vi "Get Chan Data for typedefs.vi"(7 "Custom Device Ref":T1=18446744073709551615 format="%.0x", 8 "error in":errorcluster, 10 "Ctl Ref":refnum<vi>, 11 "Section Ref in":T1 format="%.0x") -> (0 "error out":errorcluster, 2 "Indexes":i32[](array[numeric]), 3 "Section Ref out":T1 format="%.0x")   [LabVIEW 2016, in "DCM System Explorer.lvlib"]
uses:
  DCM System Explorer.lvlib
  <vilib>/NI Veristand/Custom Device API/Custom Device Item Ref.ctl
  <vilib>/NI VeriStand/Custom Device API/Custom Device API.lvlib
  <vilib>/NI Veristand/Custom Device Tools/Custom Device Utility Library/Custom Device Utility Library.lvlib
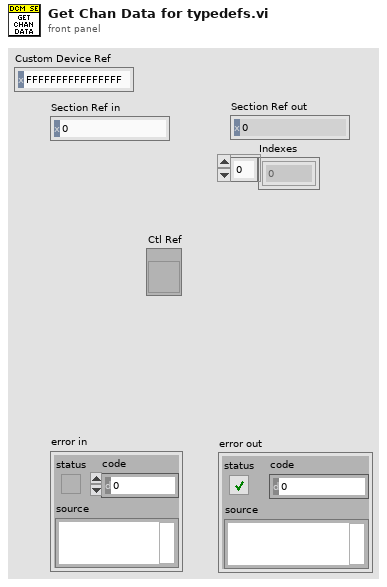
[diagram p1: front panel]
types:
  T1 = typedef "Custom Device API.lvlib/Custom Device Item Ref.ctl" = u64
  T2 = cluster{"Index Ref":refnum<vi>, "Array Refs":refnum<vi>[], "Array Positions":i32[][], "Device Ref":T1, "Section Ref":T1, "GUIDChDelProt":string, "GUIDSectDelProt":string}
  T3 = cluster{"Index Ref":refnum<vi>, "Array Refs":refnum<vi>[], "Array Positions":i32[][], "Device Ref":T1, "Section Ref":T1, "GUIDChDelProt":string, "GUIDSectDelProt":string}[]
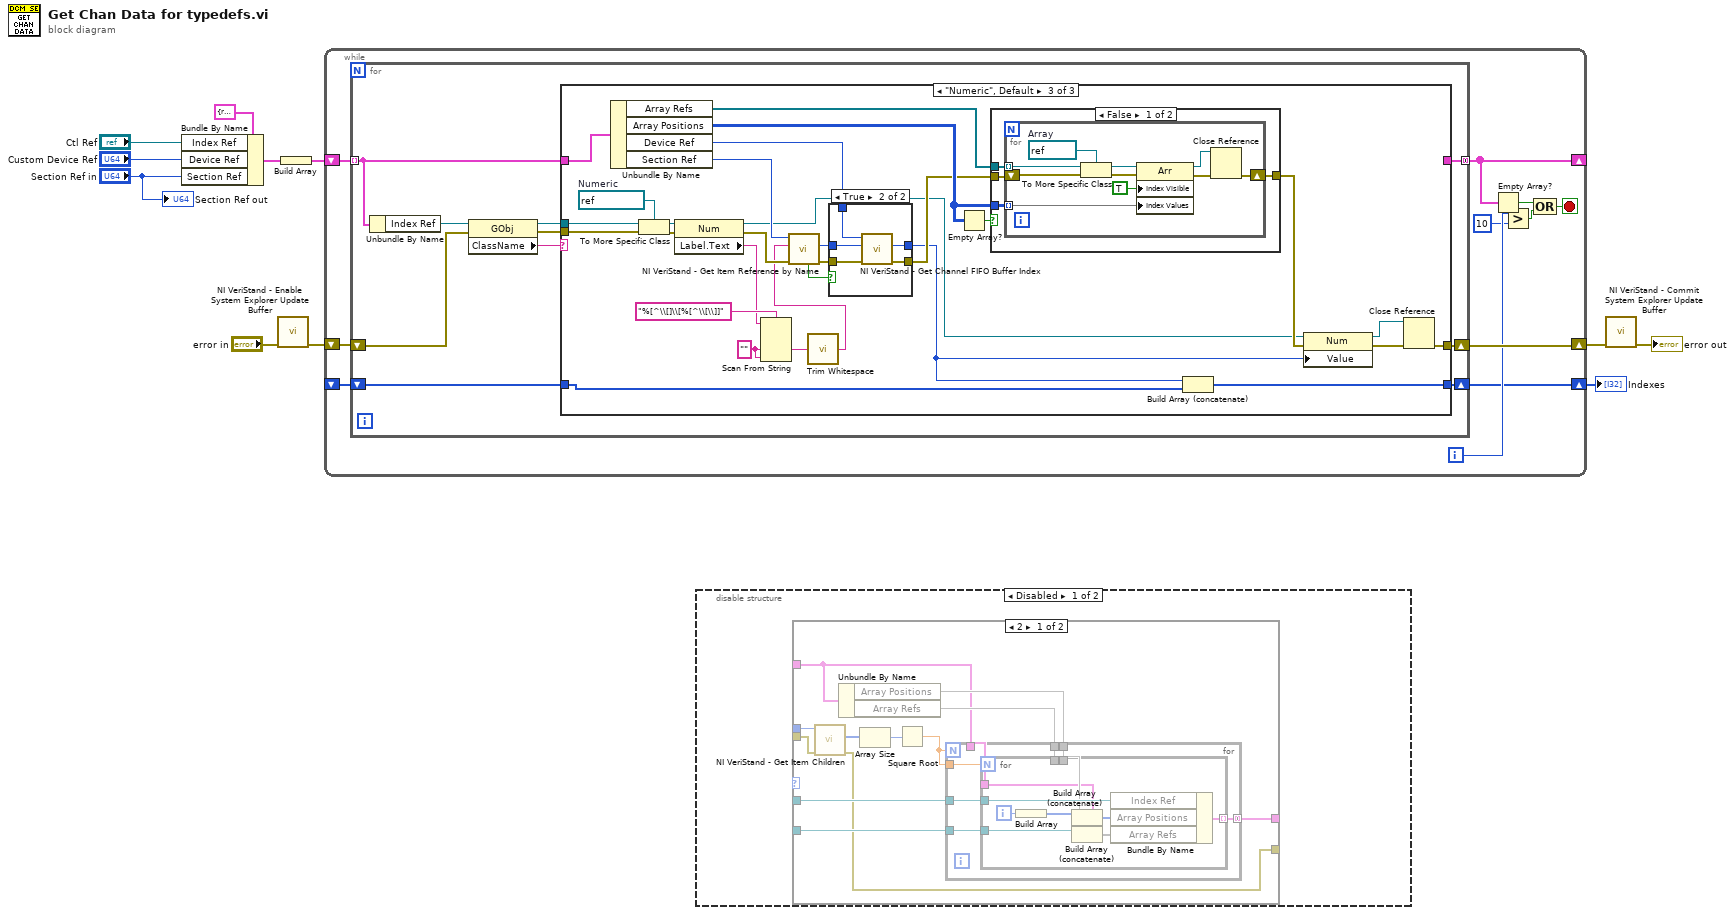
[diagram p0: block diagram]
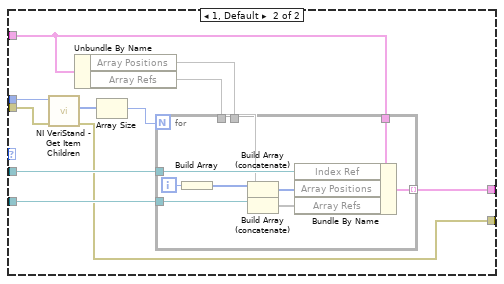
[diagram p2: hidden frame]
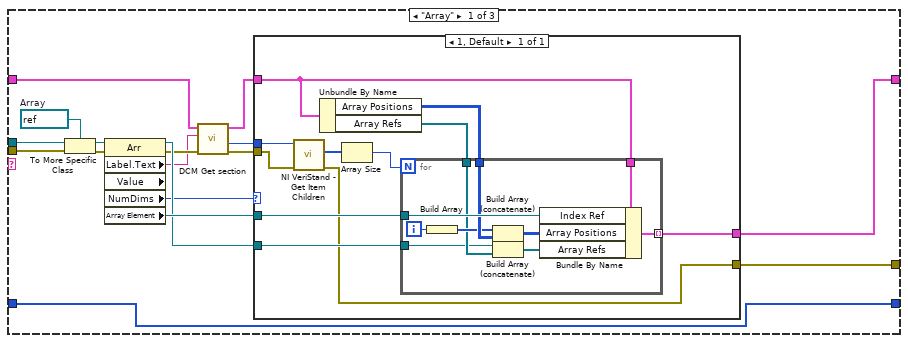
[diagram p4: hidden frame]
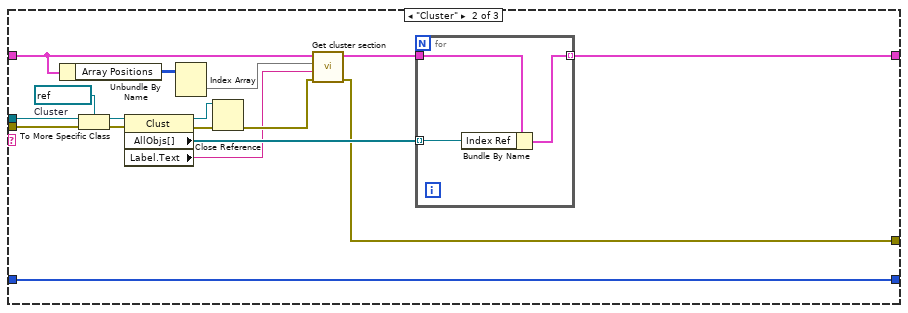
[diagram p5: hidden frame]
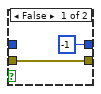
[diagram p6: hidden frame]
diagram:
  n1 = Bundle By Name(cluster=T2 {"Index Ref"=refnum, "Array Refs"=[], "Array Positions"=[], "Device Ref"=0, "Section Ref"=0, "GUIDChDelProt"="", "GUIDSectDelProt"=""} ("Data"), "Index Ref"="Ctl Ref", "Device Ref"="Custom Device Ref", "Section Ref"="Section Ref in") -> (w10:T2)
  n2 = call <vilib>:"NI VeriStand - Enable System Explorer Update Buffer.vi"("error in (no error)"="error in") -> ("error out"=w2:errorcluster)  [unwired: 10 in]
  n3 = Build Array(w10) -> (w11:T3)
  n4 = while {
    shift-right: [w21] -> _
    shift-left: w11 -> [w22]
    shift-right: [w20] -> w5
    shift-left: w2 -> [w19]
    shift-right: [w13] -> w1
    shift-left: _ -> [w12]
    i -> [w16]
    stop <- w17 stop-if-true
    n5 = for {
      tunnel: w22 -> [w29] mode=indexing
      tunnel: [w25] -> w21 mode=concatenating
      shift-right: [w30] -> w20
      shift-left: w19 -> [w26]
      shift-right: [w24] -> w13
      shift-left: w12 -> [w23]
      n6 = Unbundle By Name(w29) -> ("Index Ref"=w31:refnum<vi>)
      n7 = property class="GObj"(reference=w31, error in=w26) -> (reference out=w32:refnum<vi>, error out=w27:errorcluster, "ClassName"=w28:string)
      n8 = case shown="\"Numeric\", Default" w28 {
        tunnel: w32 -> [w49 w85 w119]
        tunnel: w27 -> [w46 w84 w117]
        tunnel: [w43 w73 w105] -> w30
        tunnel: w29 -> [w41 w77 w116]
        tunnel: [w44 w78 _] -> w25
        tunnel: [w33 w71 w91] -> w24
        tunnel: w23 -> [w33 w71 w92]
        frame "Array" {
          w45 = refnum<vi> refnum  # Array
          n9 = To More Specific Class(target class=w45, reference=w49, error in=w46) -> (specific class reference=w48:refnum<vi>, error out=w47:errorcluster)
          n10 = property class="Arr" props=["Label", "Text", "Value", "NumDims", "Array Element"](reference=w48, error in=w47) -> (reference out=w38:refnum<vi>, error out=w37:errorcluster, "Label.Text"=w36:string, "NumDims"=w34:u32, "Array Element"=w42:refnum<vi>)  [unwired: 1 out]
          n11 = call "DCM Get section.vi"("error in"=w37, "Label.Text in"=w36, "Data in"=w41) -> ("error out"=w39:errorcluster, "Section Ptr"=w35:T1, "Data out"=w40:T2)  [unwired: 6 in]
          n12 = case shown="1, Default" w34 {
            tunnel: w39 -> [w50]
            tunnel: w40 -> [w56]
            tunnel: [w60] -> w44
            tunnel: [w53] -> w43
            tunnel: w42 -> [w59]
            tunnel: w38 -> [w55]
            tunnel: w35 -> [w51]
            frame 1, Default {
              n13 = call <vilib>:"NI VeriStand - Get Item Children.vi"("error in (no error)"=w50, "Item Ref in"=w51) -> ("error out"=w53:errorcluster, "Child Refs"=w54:T1[])  [unwired: 6 in, 2 out]
              n14 = Unbundle By Name(w56) -> ("Array Positions"=w58:i32[][], "Array Refs"=w57:refnum<vi>[])
              n15 = Array Size(array=w54) -> (size(s)=w52:i32)
              n16 = for {
                N: w52 -> [_]
                tunnel: w56 -> [w70]
                tunnel: [w69] -> w60 mode=indexing
                tunnel: w59 -> [w67]
                tunnel: w55 -> [w61]
                tunnel: w58 -> [w64]
                tunnel: w57 -> [w62]
                i -> [w68]
                n17 = Build Array(w68) -> (w63:i32[])
                n18 = Build Array (concatenate)(w63, w64) -> (w66:i32[][])
                n19 = Build Array (concatenate)(w61, w62) -> (w65:refnum<vi>[])
                n20 = Bundle By Name(cluster=w70, "Index Ref"=w67, "Array Positions"=w66, "Array Refs"=w65) -> (w69:T2)
              }
            }
          }
        }
        frame "Cluster" {
          w83 = refnum<vi> refnum  # Cluster
          n21 = Unbundle By Name(w77) -> ("Array Positions"=w81:i32[][])
          n22 = To More Specific Class(target class=w83, reference=w85, error in=w84) -> (specific class reference=w87:refnum<vi>, error out=w86:errorcluster)
          n23 = property class="Clust"(reference=w87, error in=w86) -> (reference out=w80:refnum<vi>, error out=w79:errorcluster, "AllObjs[]"=w82:refnum<vi>[], "Label.Text"=w72:string)
          n24 = Index Array(array=w81) -> (element=w76:i32[])  [unwired: 2 in]
          n25 = Close Reference(reference=w80, error in (no error)=w79) -> (error out=w74:errorcluster)
          n26 = call "Get cluster section.vi"("error in (no error)"=w74, "Name (none)"=w72, "Array Positions (none)"=w76, "Data in"=w77) -> ("error out"=w73:errorcluster, "Data out"=w75:T2)  [unwired: 4 in, 2 out]
          n27 = for {
            tunnel: w75 -> [w89]
            tunnel: w82 -> [w88] mode=indexing
            tunnel: [w90] -> w78 mode=indexing
            n28 = Bundle By Name(cluster=w89, "Index Ref"=w88) -> (w90:T2)
          }
        }
        frame "Numeric", Default {
          w104 = "" ("default value 2")
          w114 = refnum<vi> refnum  # Numeric
          n29 = Unbundle By Name(w116) -> ("Array Refs"=w112:refnum<vi>[], "Array Positions"=w110:i32[][], "Device Ref"=w115:T1, "Section Ref"=w101:T1)
          n30 = To More Specific Class(target class=w114, reference=w119, error in=w117) -> (specific class reference=w118:refnum<vi>, error out=w113:errorcluster)
          n31 = property class="Num"(reference=w118, error in=w113) -> (reference out=w95:refnum<vi>, error out=w100:errorcluster, "Label.Text"=w94:string)
          n32 = Scan From String(format string="%[^\\[]\\[%[^\\[\\]]" ("regular expression"), input string=w94, default 1=w104, default 2=w104) -> (output 1=w103:string)  [unwired: 3 in, 3 out]
          n33 = call <vilib>:"Trim Whitespace.vi"("string"=w103) -> ("trimmed string"=w97:string)  [unwired: 1 in]
          n34 = call <vilib>:"NI VeriStand - Get Item Reference by Name.vi"("error in (no error)"=w100, "Item Name"=w97, "Parent Ref in"=w101) -> ("error out"=w99:errorcluster, "Item Ref"=w98:T1, "Found"=w96:bool)  [unwired: 5 in, 1 out]
          n35 = case shown="True" w96 {
            tunnel: w115 -> [_ w126]
            tunnel: [w121 w125] -> w109
            tunnel: [-1 ("Channel FIFO Buffer Index") w124] -> w93
            tunnel: w99 -> [w121 w123]
            tunnel: w98 -> [_ w122]
            frame False {
            }
            frame True {
              n36 = call <vilib>:"NI VeriStand - Get Channel FIFO Buffer Index.vi"("error in"=w123, "Channel Ref"=w122, "Device Ref in"=w126) -> ("error out"=w125:errorcluster, "Channel FIFO Buffer Index"=w124:i32)  [unwired: 4 in, 3 out]
            }
          }
          n37 = Empty Array?(array=w110) -> (empty?=w111:bool)
          n38 = case shown="False" w111 {
            tunnel: w112 -> [w130 _]
            tunnel: w110 -> [w129 _]
            tunnel: w109 -> [w127 w141]
            tunnel: [w128 w141] -> w108
            frame False {
              n39 = for {
                tunnel: w130 -> [w134] mode=indexing
                tunnel: w129 -> [w138] mode=indexing
                shift-right: [w131] -> w128
                shift-left: w127 -> [w136]
                w140 = refnum<vi> refnum  # Array
                n40 = To More Specific Class(target class=w140, reference=w134, error in=w136) -> (specific class reference=w139:refnum<vi>, error out=w135:errorcluster)
                n41 = property class="Arr"(reference=w139, error in=w135, "Index Visible"=TRUE, "Index Values"=w138) -> (reference out=w132:refnum<vi>, error out=w133:errorcluster)
                n42 = Close Reference(reference=w132, error in (no error)=w133) -> (error out=w131:errorcluster)
              }
            }
            frame True {
            }
          }
          n43 = Build Array (concatenate)(w93, w92) -> (w91:i32[])
          n44 = property class="Num"(reference=w95, error in=w108, "Value"=w93) -> (reference out=w106:refnum<vi>, error out=w107:errorcluster)
          n45 = Close Reference(reference=w106, error in (no error)=w107) -> (error out=w105:errorcluster)
        }
      }
    }
    n46 = Empty Array?(array=w21) -> (empty?=w18:bool)
    n47 = Greater?(x=w16, y=10) -> (0:w14:bool)
    n48 = Compound Arithmetic op=OR(w18, w14) -> (w17:bool)
  }
  "Indexes" <- w1
  n49 = disable-structure shown="Disabled" {
    frame Disabled {
      n50 = case shown="2" {
        selector: _ -> [_ _]
        tunnel: _ -> [w146 w171]
        tunnel: _ -> [w149 w177]
        tunnel: [w153 w181] -> _
        tunnel: [w144 w174] -> _
        tunnel: _ -> [w152 w180]
        tunnel: _ -> [w148 w176]
        tunnel: _ -> [w147 w172]
        frame 2 {
          n51 = call <vilib>:"NI VeriStand - Get Item Children.vi"("error in (no error)"=w146, "Item Ref in"=w147) -> ("error out"=w144:errorcluster, "Child Refs"=w145:T1[])  [unwired: 6 in, 2 out]
          n52 = Unbundle By Name(w149) -> ("Array Positions"=w151, "Array Refs"=w150)
          n53 = Array Size(array=w145) -> (size(s)=w143:i32)
          n54 = Square Root(x=w143) -> (sqrt(x)=w142:dbl)
          n55 = for {
            N: w142 -> [_]
            tunnel: w142 -> [w160]
            tunnel: [w158] -> w153 mode=concatenating
            tunnel: w152 -> [w159]
            tunnel: w148 -> [w157]
            tunnel: w151 -> [w156]
            tunnel: w150 -> [w155]
            tunnel: w149 -> [w154]
            n56 = for {
              N: w160 -> [_]
              tunnel: w159 -> [w168]
              tunnel: [w169] -> w158 mode=indexing
              tunnel: w157 -> [w164]
              tunnel: w156 -> [w163]
              tunnel: w155 -> [w165]
              tunnel: w154 -> [w161]
              i -> [w170]
              n57 = Build Array(w170) -> (w162:i32[])
              n58 = Build Array (concatenate)(w162, w163) -> (w167:i32[])
              n59 = Build Array (concatenate)(w164, w165) -> (w166:void[])
              n60 = Bundle By Name(cluster=w161, "Index Ref"=w168, "Array Positions"=w167, "Array Refs"=w166) -> (w169:cluster{})
            }
          }
        }
        frame 1, Default {
          n61 = call <vilib>:"NI VeriStand - Get Item Children.vi"("error in (no error)"=w171, "Item Ref in"=w172) -> ("error out"=w174:errorcluster, "Child Refs"=w175:T1[])  [unwired: 6 in, 2 out]
          n62 = Unbundle By Name(w177) -> ("Array Positions"=w179, "Array Refs"=w178)
          n63 = Array Size(array=w175) -> (size(s)=w173:i32)
          n64 = for {
            N: w173 -> [_]
            tunnel: w177 -> [w191]
            tunnel: [w190] -> w181 mode=indexing
            tunnel: w180 -> [w188]
            tunnel: w176 -> [w182]
            tunnel: w179 -> [w185]
            tunnel: w178 -> [w183]
            i -> [w189]
            n65 = Build Array(w189) -> (w184:i32[])
            n66 = Build Array (concatenate)(w184, w185) -> (w187:i32[])
            n67 = Build Array (concatenate)(w182, w183) -> (w186:void[])
            n68 = Bundle By Name(cluster=w191, "Index Ref"=w188, "Array Positions"=w187, "Array Refs"=w186) -> (w190:cluster{})
          }
        }
      }
    }
    frame Enabled {
    }
  }
  n69 = call <vilib>:"NI VeriStand - Commit System Explorer Update Buffer.vi"("error in (no error)"=w5) -> ("error out"=→"error out":errorcluster)  [unwired: 10 in]
  "Section Ref out" <- "Section Ref in"
